vi "qWTR.vi"(0 "System no.":i32=1 min=1 max=4 step=1, 2 "Generator ID to query":i32[](array[numeric]) min=1 step=1, 3 "All Generator IDs?":bool, 5 "error in":errorcluster) -> (14 "Table rate":i32[](array[numeric]), 15 "Interpolation type":i32[](array[numeric]), 19 "error out":errorcluster)   [LabVIEW 2026]
doc: "Returns the current settings of the wave generator table rate.\n\nC-413 : Generator ID can be 1 to 2\n\nC-886: Values quried for one Generator ID are valid for all generators.\n\nC-887: Values quried for one Generator ID are valid for all generators. \n\nC-891: Generator ID can be 1.\n\nE-517, E-518: Generator ID can be 1 to 3. \n\nE-709: Generator ID can be 0 or 1 because there is only one generator. \n\nE-712: Generator ID must be 0 because values are valid for all generators.\n\nE-725, E-727: Generator ID must be 0 because values are valid for all generators.\n\nE-753: Generator ID must be 0 because values are valid for all generators.\n\nE-754: Generator ID must be 0 because values are valid for all generators."
panel:
  # "Returns the current settings of the wave generator table rate."
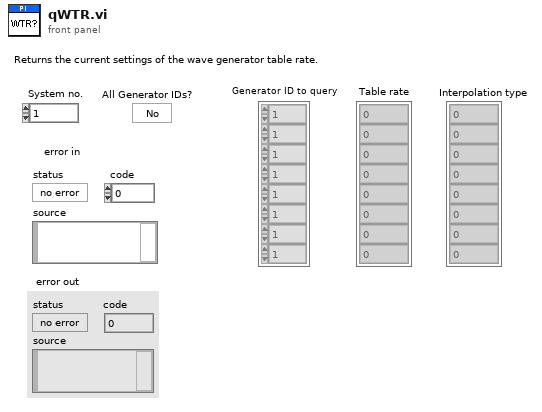
[diagram p1: front panel]
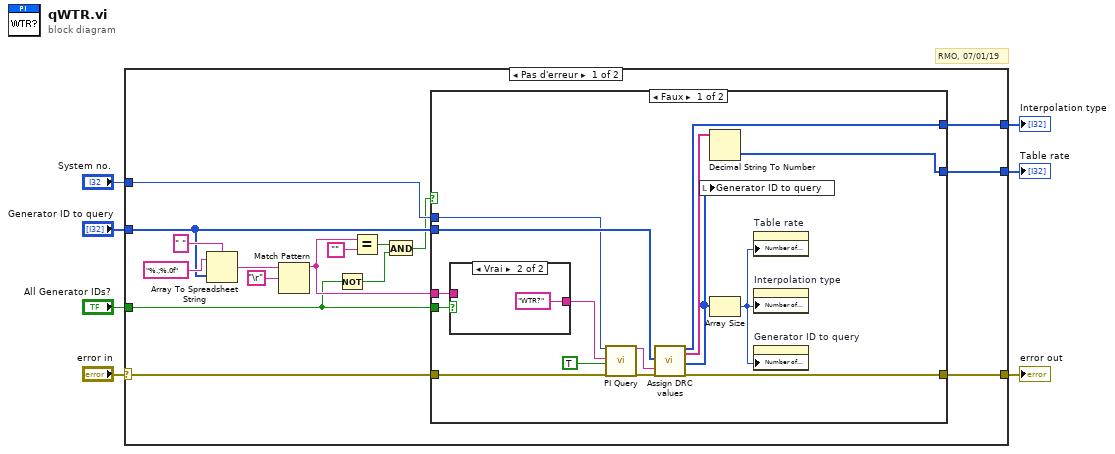
[diagram p0: block diagram]
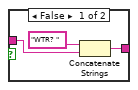
[diagram p2: hidden frame]
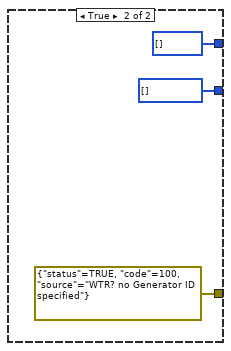
[diagram p3: hidden frame]
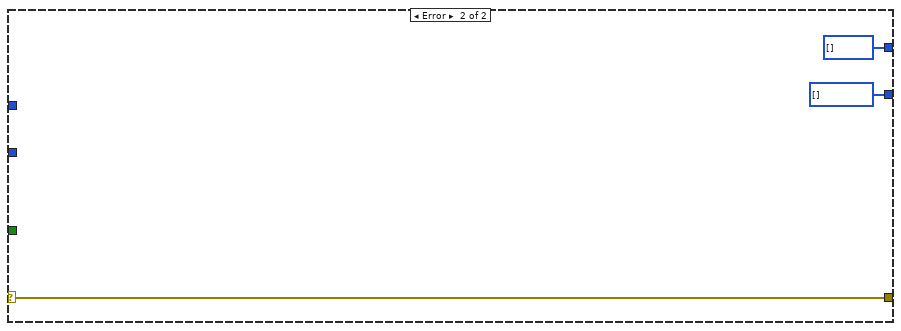
[diagram p4: hidden frame]
diagram:
  # "RMO, 07/01/19"
  n1 = case shown="Pas d'erreur" "error in" {
    selector: "error in" -> [w8 w46]
    tunnel: "Generator ID to query" -> [w14 _]
    tunnel: "System no." -> [w20 _]
    tunnel: [w22 w46] -> w5
    tunnel: [w21 i32[] [] ("Parameter values")] -> w4
    tunnel: [w15 i32[] [] ("Source ID")] -> w3
    tunnel: "All Generator IDs?" -> [w10 _]
    frame No Error {
      n2 = Array To Spreadsheet String(delimiter (Tab)=" ", array=w14, 3:"%.;%.0f" ("Format String")) -> (spreadsheet string=w16:string)
      n3 = Match Pattern(string=w16, regular expression="\r") -> (before substring=w13:string)  [unwired: 4 out]
      n4 = Not(x=w10) -> (.not. x?=w9:bool)
      n5 = Equal?(x=w13, y="" ("x")) -> (x = y?=w11:bool)
      n6 = And(x=w11, y=w9) -> (x .and. y?=w12:bool)
      n7 = case shown="Faux" w12 {
        tunnel: w8 -> [w35 _]
        tunnel: w13 -> [w36 _]
        tunnel: w20 -> [w32 _]
        tunnel: [w34 errorcluster {"status"=TRUE, "code"=100, "source"="WTR? no Generator ID specified"} ("error out")] -> w22
        tunnel: [w28 i32[] [] ("Parameter values")] -> w21
        tunnel: [w26 i32[] [] ("Source ID")] -> w15
        tunnel: w14 -> [w33 _]
        tunnel: w10 -> [w31 _]
        frame False {
          n8 = case shown="Vrai" w31 {
            tunnel: [w40 "WTR?"] -> w37
            tunnel: w36 -> [w39 _]
            frame False {
              n9 = Concatenate Strings("WTR? ", w39) -> (w40:string)
            }
            frame True {
            }
          }
          n10 = call "PI Query.vi"("System no."=w32, "String to send"=w37, "Attach termination char.?"=TRUE ("Attach Linefeed?"), "error in"=w35) -> ("String read"=w24:string, "error out"=w25:errorcluster)  [unwired: 3 in, 11 out]
          n11 = call "Assign DRC values.vi"("Queried Rec. table"=w33, "Input String"=w24, "error in"=w25) -> ("Rec. option"=w26:i32[], "Source ID"=w29:string[], "Queried Rec. table out"=w30:i32[], "error out"=w34:errorcluster)  [unwired: 1 in, 12 out]
          n12 = local write "Generator ID to query"(w30) -> ()
          n13 = Decimal String To Number(string=w29) -> (number=w28:i32[])  [unwired: 3 out]
          n14 = Array Size(array=w30) -> (size(s)=w27:i32)
          n15 = property on="Table rate" class="Tabl (strict)"("Number of Rows"=w27) -> ()  [unwired: 2 in, 2 out]
          n16 = property on="Interpolation type" class="Tabl (strict)"("Number of Rows"=w27) -> ()  [unwired: 2 in, 2 out]
          n17 = property on="Generator ID to query" class="Tabl (strict)"("Number of Rows"=w27) -> ()  [unwired: 2 in, 2 out]
        }
        frame True {
        }
      }
    }
    frame Error {
    }
  }
  "Interpolation type" <- w3
  "error out" <- w5
  "Table rate" <- w4
